vi "Shift Window.vi"(8 "error in (no error)":errorcluster, 10 "top left point":cluster{"x":i16, "y":i16}, 11 "ViewableActor in":refnum<class "ViewableActor.lvclass">) -> (0 "error out":errorcluster, 3 "ViewableActor out":refnum<class "ViewableActor.lvclass">)   [LabVIEW 2020, in "ViewableActor.lvlib" / "ViewableActor.lvclass"]
uses:
  ViewableActor.lvclass
  ViewableActor.lvclass/ViewableActor.ctl
  Read UI VI Ref.vi
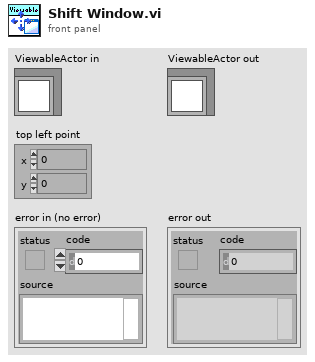
[diagram p1: front panel]
types:
  T1 = typedef "LVRectTypeDef.ctl" = cluster{"Left":i16, "Top":i16, "Right":i16, "Bottom":i16}
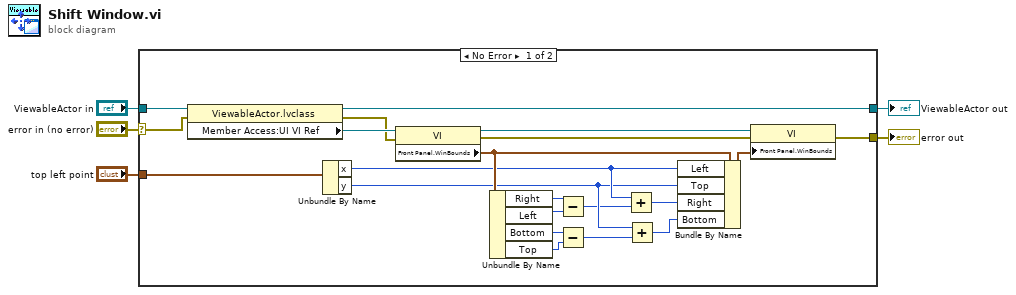
[diagram p0: block diagram]
diagram:
  n1 = case shown="No Error" "error in (no error)" {
    selector: "error in (no error)" -> [w21 w28]
    tunnel: [w6 w28] -> w4
    tunnel: [w24 w27] -> w2
    tunnel: "ViewableActor in" -> [w26 w27]
    tunnel: "top left point" -> [w25 _]
    frame No Error {
      n2 = property class="ViewableActor.lvclass"(reference=w26, error in=w21) -> (reference out=w24:refnum<class "ViewableActor.lvclass">, error out=w22:errorcluster, "Member Access:UI VI Ref"=w23:refnum<vi>)
      n3 = Unbundle By Name(w25) -> ("x"=w10:i16, "y"=w8:i16)
      n4 = property class="VI"(reference=w23, error in=w22) -> (reference out=w20:refnum<vi>, error out=w19:errorcluster, "Front Panel.WinBounds"=w17:T1)
      n5 = Unbundle By Name(w17) -> ("Right"=w16:i16, "Left"=w15:i16, "Bottom"=w14:i16, "Top"=w13:i16)
      n6 = Subtract(x=w16, y=w15) -> (x-y=w7:i16)
      n7 = Subtract(x=w14, y=w13) -> (x-y=w12:i16)
      n8 = Add(x=w10, y=w7) -> (x+y=w9:i16)
      n9 = Add(x=w8, y=w12) -> (x+y=w11:i16)
      n10 = Bundle By Name(cluster=w17, "Left"=w10, "Top"=w8, "Right"=w9, "Bottom"=w11) -> (w18:T1)
      n11 = property class="VI"(reference=w20, error in=w19, "Front Panel.WinBounds"=w18) -> (error out=w6:errorcluster)  [unwired: 1 out]
    }
    frame Error {
    }
  }
  "error out" <- w4
  "ViewableActor out" <- w2
